vi "Partition_Format.vi"(9 "Grid":string[][](array[string]), 10 "Data":string[][](array[string]), 11 "Labels in":string[](array[string])=["Partition", "A", "B", "C", "D", "E", "F", "G", "X", "", "", "", "", "", "", "", "", ""]) -> (1 "Array 3":string[](array[string]), 2 "Alphabetical":string[](array[string]), 3 "Grid out":string[][](array[string]), 4 "Labels out":string[](array[string]), 5 "empty Element":string[](array[string]))   [LabVIEW 2020]
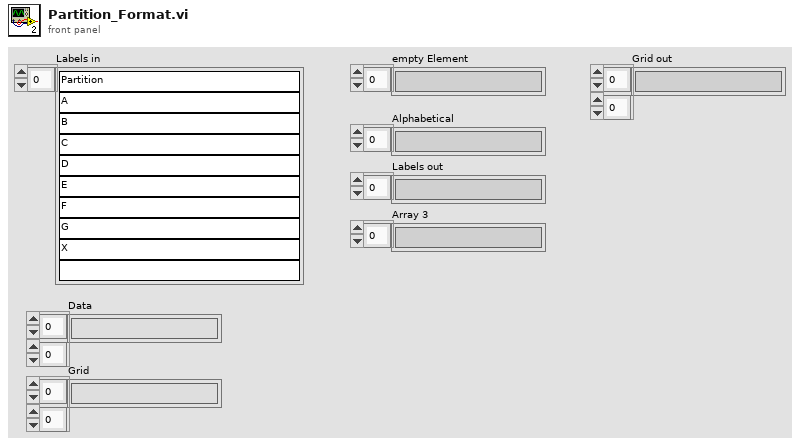
[diagram p1: front panel]
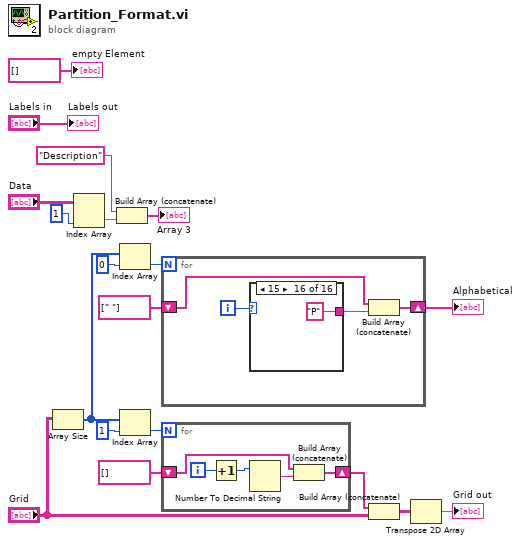
[diagram p0: block diagram]
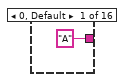
[diagram p2: hidden frame]
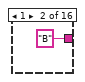
[diagram p3: hidden frame]
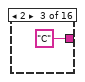
[diagram p4: hidden frame]
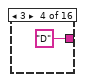
[diagram p5: hidden frame]
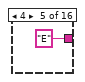
[diagram p6: hidden frame]
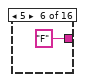
[diagram p7: hidden frame]
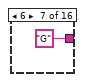
[diagram p8: hidden frame]
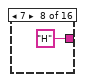
[diagram p9: hidden frame]
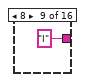
[diagram p10: hidden frame]
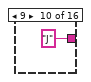
[diagram p11: hidden frame]
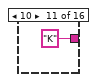
[diagram p12: hidden frame]
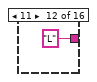
[diagram p13: hidden frame]
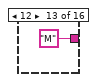
[diagram p14: hidden frame]
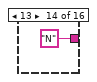
[diagram p15: hidden frame]
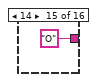
[diagram p16: hidden frame]
diagram:
  n1 = Array Size(array="Grid") -> (size(s)=w13:i32[])
  n2 = Index Array(array="Data", index (col)=1 ("disabled index (col)")) -> (element=w4:string[])  [unwired: 1 in]
  n3 = Build Array (concatenate)("Description" ("element"), w4) -> (→"Array 3":string[])
  n4 = Index Array(array=w13, index=0) -> (element=w16:i32)
  n5 = Index Array(array=w13, index=1) -> (element=w9:i32)
  n6 = for {
    N: w16 -> [_]
    shift-right: [w21] -> w17
    shift-left: string[] [" "] -> [w20]
    i -> [w23]
    n7 = case shown="15" w23 {
      tunnel: ["A" "B" "C" "D" "E" "F" "G" "H" "I" "J" "K" "L" "M" "N" "O" "P"] -> w22
      frame 0, Default {
      }
      frame 1 {
      }
      frame 2 {
      }
      frame 3 {
      }
      frame 4 {
      }
      frame 5 {
      }
      frame 6 {
      }
      frame 7 {
      }
      frame 8 {
      }
      frame 9 {
      }
      frame 10 {
      }
      frame 11 {
      }
      frame 12 {
      }
      frame 13 {
      }
      frame 14 {
      }
      frame 15 {
      }
    }
    n8 = Build Array (concatenate)(w20, w22) -> (w21:string[])
  }
  "Alphabetical" <- w17
  n9 = for {
    N: w9 -> [_]
    shift-right: [w40] -> w11
    shift-left: string[] [] -> [w43]
    i -> [w44]
    n10 = Increment(x=w44) -> (x+1=w42:i32)
    n11 = Number To Decimal String(number=w42) -> (decimal integer string=w41:string)  [unwired: 1 in]
    n12 = Build Array (concatenate)(w43, w41) -> (w40:string[])
  }
  n13 = Build Array (concatenate)(w11, "Grid") -> (w18:string[][])
  n14 = Transpose 2D Array(2D array=w18) -> (transposed array=→"Grid out":string[][])
  "Labels out" <- "Labels in"
  "empty Element" <- string[] [] ("element")
